vi "InitFFT_Buffer.vi"(6 "FFT buffer size":T1, 8 "error in (no error)":errorcluster, 9 "dimension size":i32=7, 10 "Transfer speed":T2, 11 "ScopeBase In":refnum<class "ScopeBase.lvclass">) -> (0 "error out":errorcluster, 3 "ScopeBase Out":refnum<class "ScopeBase.lvclass">)   [LabVIEW 2025, in "ScopeBase.lvclass"]
uses:
  ScopeBase.lvclass
  controls/host_transfer_speed.ctl
  controls/FFT buffer type.ctl
  ScopeBase.lvclass/ScopeBase.ctl
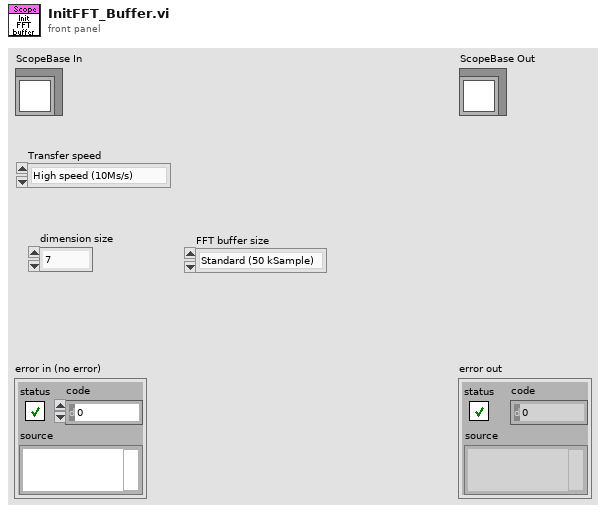
[diagram p1: front panel]
types:
  T1 = typedef "FFT buffer type.ctl" = enum16{"Standard (50 kSample)", "Long (250 kSample)"}
  T2 = typedef "host_transfer_speed.ctl" = enum16{"High speed (10Ms/s)", "Low speed (1Ms/s)", "Ultra low speed (50kS/s)"}
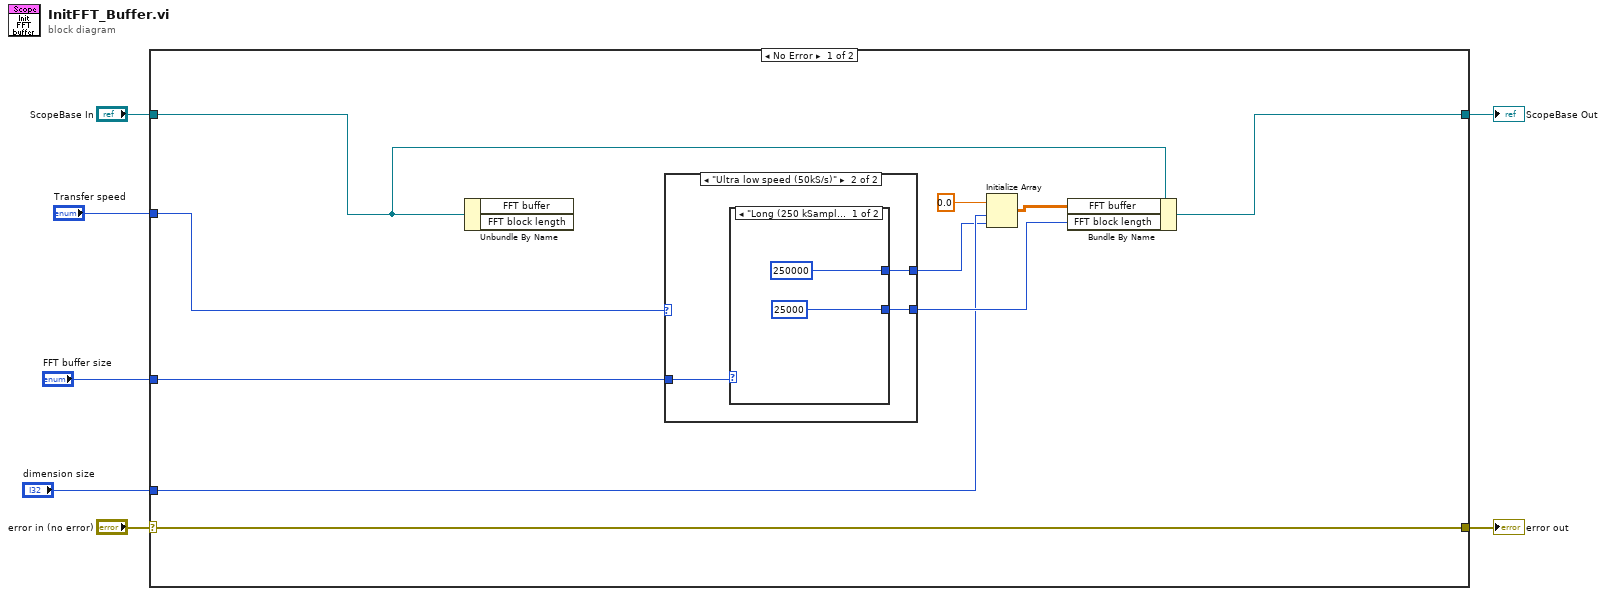
[diagram p0: block diagram]
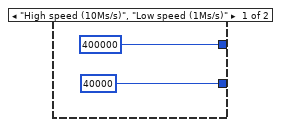
[diagram p2: hidden frame]
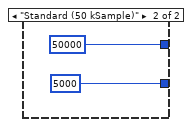
[diagram p3: hidden frame]
diagram:
  n1 = case shown="No Error" "error in (no error)" {
    selector: "error in (no error)" -> [w17 w28]
    tunnel: [w17 w28] -> w5
    tunnel: [w16 w27] -> w6
    tunnel: "ScopeBase In" -> [w15 w27]
    tunnel: "Transfer speed" -> [w14 _]
    tunnel: "dimension size" -> [w10 _]
    tunnel: "FFT buffer size" -> [w8 _]
    frame No Error {
      n2 = Unbundle By Name(w15) -> ()  [unwired: 2 out]
      n3 = case shown="\"Ultra low speed (50kS/s)\"" w14 {
        tunnel: [400000 w22] -> w9
        tunnel: [40000 w21] -> w13
        tunnel: w8 -> [_ w20]
        frame "High speed (10Ms/s)", "Low speed (1Ms/s)" {
        }
        frame "Ultra low speed (50kS/s)" {
          n4 = case shown="\"Long (250 kSample)\"" w20 {
            tunnel: [250000 50000] -> w22
            tunnel: [25000 5000] -> w21
            frame "Long (250 kSample)" {
            }
            frame "Standard (50 kSample)" {
            }
          }
        }
      }
      n5 = Initialize Array(0.0, w10, w9) -> (w11:dbl[][])
      n6 = Bundle By Name(cluster=w15, "FFT buffer"=w11, "FFT block length"=w13) -> (w16:refnum<class "ScopeBase.lvclass">)
    }
    frame Error {
    }
  }
  "error out" <- w5
  "ScopeBase Out" <- w6
